vi "DriftInPixel (SubVI).vi"(10 "New image":dbl[][](array[numeric]), 11 "Ref image":dbl[][](array[numeric])) -> (0 "pixel":i32, 2 "Y drift":i32, 3 "X drift":i32)   [LabVIEW 2014]
uses:
  <vilib>/Analysis/2dsp.llb/2D Cross Correlation (DBL).vi
  <vilib>/Analysis/NI_AALPro.lvlib
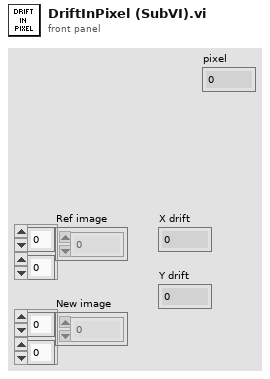
[diagram p1: front panel]
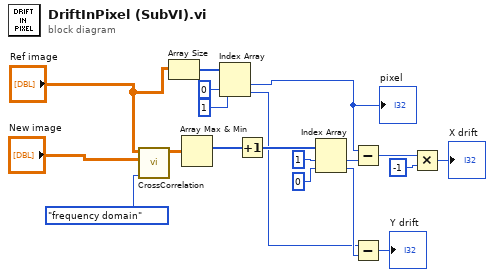
[diagram p0: block diagram]
diagram:
  n1 = call-poly <vilib>:"CrossCorrelation.vi"("algorithm"=enum32{"direct", "frequency domain"}."frequency domain", "Y"="New image", "X"="Ref image") -> ("Rxy"=w7:dbl[][])  [unwired: 7 in, 1 out]
  n2 = Array Size(array="Ref image") -> (size(s)=w5:i32[])
  n3 = Array Max & Min(array=w7) -> (max index (indices)=w18:i32[])  [unwired: 3 out]
  n4 = Index Array(array=w5, index #1=0 ("index"), index #2=1 ("index")) -> (element #1=w2:i32, element #2=w1:i32)
  "pixel" <- w2
  n5 = Increment(x=w18) -> (x+1=w19:i32[])
  n6 = Index Array(array=w19, index #1=1 ("index"), index #2=0 ("index")) -> (element #1=w11:i32, element #2=w12:i32)
  n7 = Subtract(x=w2, y=w11) -> (x-y=w13:i32)
  n8 = Subtract(x=w1, y=w12) -> (x-y=→"Y drift":i32)
  n9 = Multiply(x=w13, y=-1) -> (x*y=→"X drift":i32)
